vi "Convert2user units.vi"(0 "Configration.Table":T3[](array[typedef]), 1 "Lens Property In":T1={"Unit"=TRUE, "Start "=1.0, "Stop "=1.0, "Dwell Time"=1.0, "Pause Time"=1.0, "Scans"=1, "Step Size"=1.0, "Row Numer"=0, "Ramp Time (ms)"=1, "Start DAC"=0, "Scan Type"=enum."Single"}, 2 "error in (no error)":errorcluster) -> (3 "OP 1":dbl, 4 "OP 2":dbl, 5 "OP 3":dbl, 6 "error out":errorcluster)   [LabVIEW 2018]
uses:
  GC-MSMSDevlopment/Type/_RT Configuration 2.ctl
  Type Defs/Lens Property.ctl
  Type Defs/Scan Type.ctl
  Type Defs/Global Action.ctl
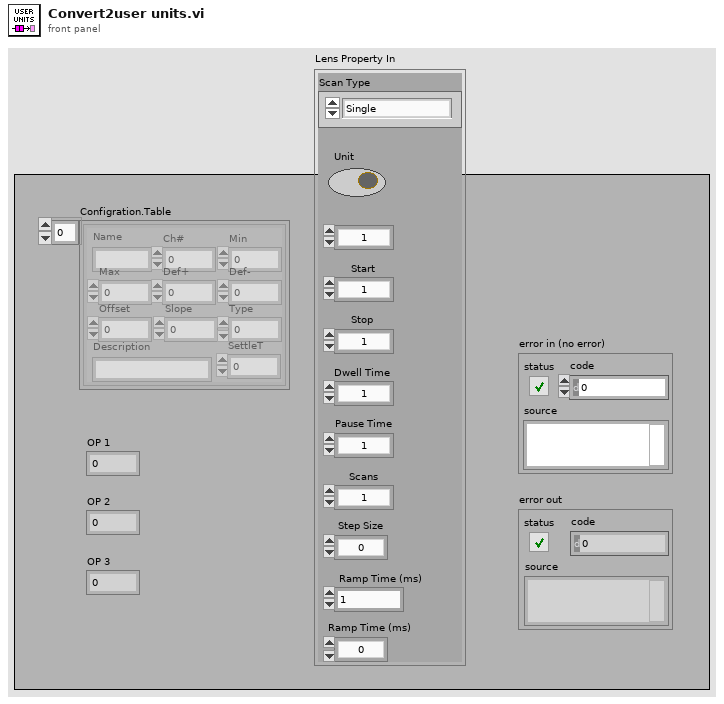
[diagram p1: front panel]
types:
  T1 = typedef "Lens Property.ctl" = cluster{"Unit":bool, "Start ":dbl, "Stop ":dbl, "Dwell Time":dbl, "Pause Time":dbl, "Scans":i32, "Step Size":dbl, "Row Numer":i32, "Ramp Time (ms)":i32, "Start DAC":i32, "Scan Type":T2}
  T2 = typedef "Scan Type.ctl" = enum8{"Single", "Dual", "Ramp"}
  T3 = typedef "_RT Configuration 2.ctl" = cluster{"Name":string, "Ch#":u8, "Min":dbl, "Max":dbl, "Def+":dbl, "Def-":dbl, "Offset":dbl, "Slope":dbl, "Type":u8, "Description":string, "SettleT":dbl}
  T4 = typedef "Global Action.ctl" = enum16{"Write", "Read"}
  T5 = typedef "Global Parameters.ctl" = cluster{"Calibrations":cluster{"Q1 +ve":dbl[][], "Q2 +ve":dbl[][], "Q1 -ve":dbl[][], "Q2 -ve":dbl[][]}, "Resolution Q1":cluster{"High +ve":dbl[][], "Med +ve":dbl[][], "Low +ve":dbl[][], "High -ve":dbl[][], "Med -ve":dbl[][], "Low -ve":dbl[][]}, "Resolution Q2":cluster{"High +ve":dbl[][], "Med +ve":dbl[][], "Loe +ve":dbl[][], "High -ve":dbl[][], "Med -ve":dbl[][], "Low -ve":dbl[][]}, "MR Parameters":T6, "Mass":dbl[][], "Dwell":dbl[][], "Steps":i32[][], "Method Refnum":refnum<vi>}
  T6 = typedef "MR Parameters.ctl" = cluster{"Name":string, "Ch#":u8, "StartV":dbl, "StopV":dbl, "StepV":dbl, "Index":u8}
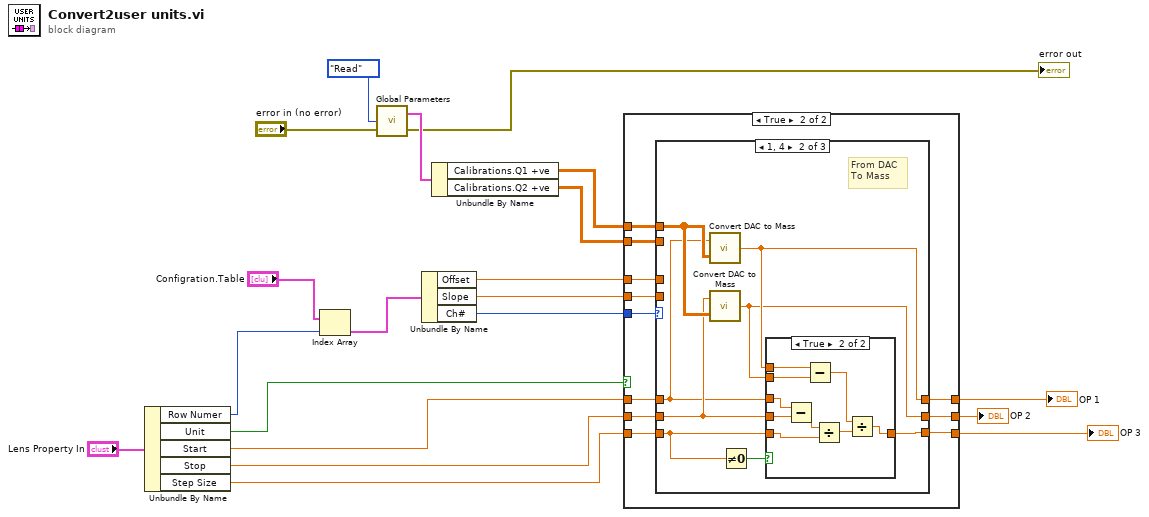
[diagram p0: block diagram]
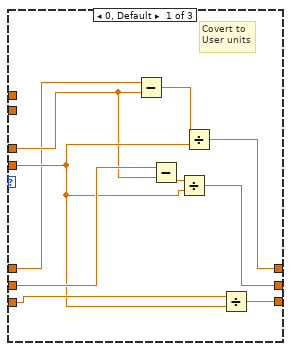
[diagram p3: hidden frame]
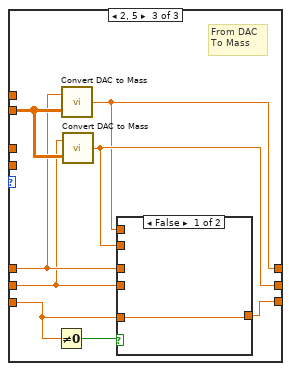
[diagram p5: hidden frame]
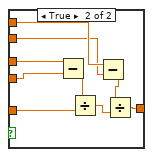
[diagram p6: hidden frame]
diagram:
  n1 = Unbundle By Name("Lens Property In") -> ("Row Numer"=w11:i32, "Unit"=w10:bool, "Start"=w9:dbl, "Stop"=w8:dbl, "Step Size"=w7:dbl)
  n2 = Index Array(array="Configration.Table", index=w11) -> (element=w17:T3)
  n3 = call "Global Parameters.vi"("Error In"="error in (no error)", "Action"=Global_Action."Read") -> ("Error Out"=→"error out":errorcluster, "Parameters Out"=w6:T5)  [unwired: 1 in]
  n4 = Unbundle By Name(w17) -> ("Offset"=w13:dbl, "Slope"=w14:dbl, "Ch#"=w15:u8)
  n5 = Unbundle By Name(w6) -> ("Calibrations.Q1 +ve"=w3:dbl[][], "Calibrations.Q2 +ve"=w4:dbl[][])
  n6 = case shown="True" w10 {
    tunnel: w9 -> [w23 w30]
    tunnel: w8 -> [w22 w31]
    tunnel: w7 -> [w21 w33]
    tunnel: w15 -> [_ w34]
    tunnel: w14 -> [_ w29]
    tunnel: w13 -> [_ w28]
    tunnel: [w23 w26] -> w20
    tunnel: [w22 w27] -> w19
    tunnel: [w21 w32] -> w18
    tunnel: w4 -> [_ w24]
    tunnel: w3 -> [_ w25]
    frame False {
    }
    frame True {
      n7 = case shown="1, 4" w34 {
        tunnel: w33 -> [w42 w50 w63]
        tunnel: [w41 w49 w69] -> w32
        tunnel: w31 -> [w40 w48 w67]
        tunnel: w30 -> [w37 w47 w68]
        tunnel: w29 -> [w39 _ _]
        tunnel: w28 -> [w38 _ _]
        tunnel: [w36 w45 w66] -> w27
        tunnel: [w35 w46 w65] -> w26
        tunnel: w25 -> [_ w52 _]
        tunnel: w24 -> [_ _ w70]
        frame 0, Default {
          # "Covert to\nUser units"
          n8 = Subtract(x=w37, y=w38) -> (x-y=w44:dbl)
          n9 = Subtract(x=w40, y=w38) -> (x-y=w43:dbl)
          n10 = Divide(x=w43, y=w39) -> (x/y=w36:dbl)
          n11 = Divide(x=w44, y=w39) -> (x/y=w35:dbl)
          n12 = Divide(x=w42, y=w39) -> (x/y=w41:dbl)
        }
        frame 1, 4 {
          # "From DAC\nTo Mass"
          n13 = call "Convert DAC to Mass.vi"("Calibration Table"=w52, "DAC"=w47) -> ("Mass"=w46:dbl)
          n14 = call "Convert DAC to Mass.vi"("Calibration Table"=w52, "DAC"=w48) -> ("Mass"=w45:dbl)
          n15 = Not Equal To 0?(x=w50) -> (x != 0?=w51:bool)
          n16 = case shown="True" w51 {
            tunnel: w50 -> [w53 w56]
            tunnel: [w53 w59] -> w49
            tunnel: w48 -> [_ w58]
            tunnel: w47 -> [_ w57]
            tunnel: w45 -> [_ w55]
            tunnel: w46 -> [_ w54]
            frame False {
            }
            frame True {
              n17 = Subtract(x=w57, y=w58) -> (x-y=w60:dbl)
              n18 = Subtract(x=w54, y=w55) -> (x-y=w61:dbl)
              n19 = Divide(x=w60, y=w56) -> (x/y=w62:dbl)
              n20 = Divide(x=w61, y=w62) -> (x/y=w59:dbl)
            }
          }
        }
        frame 2, 5 {
          # "From DAC\nTo Mass"
          n21 = Not Equal To 0?(x=w63) -> (x != 0?=w64:bool)
          n22 = call "Convert DAC to Mass.vi"("Calibration Table"=w70, "DAC"=w68) -> ("Mass"=w65:dbl)
          n23 = call "Convert DAC to Mass.vi"("Calibration Table"=w70, "DAC"=w67) -> ("Mass"=w66:dbl)
          n24 = case shown="False" w64 {
            tunnel: w63 -> [w71 w77]
            tunnel: w68 -> [_ w76]
            tunnel: w67 -> [_ w75]
            tunnel: w65 -> [_ w74]
            tunnel: w66 -> [_ w73]
            tunnel: [w71 w72] -> w69
            frame False {
            }
            frame True {
              n25 = Subtract(x=w76, y=w75) -> (x-y=w78:dbl)
              n26 = Divide(x=w78, y=w77) -> (x/y=w80:dbl)
              n27 = Subtract(x=w74, y=w73) -> (x-y=w79:dbl)
              n28 = Divide(x=w79, y=w80) -> (x/y=w72:dbl)
            }
          }
        }
      }
    }
  }
  "OP 1" <- w20
  "OP 2" <- w19
  "OP 3" <- w18
